vi "updateState.vi"(8 "error in (no error)":errorcluster, 10 "Monochromator in":refnum<class "Monochromator.lvclass">, 11 "SettingUpState in":refnum<class "SettingUpState.lvclass">) -> (0 "error out":errorcluster, 2 "Monochromator out":refnum<class "Monochromator.lvclass">, 3 "SettingUpState out":refnum<class "SettingUpState.lvclass">)   [LabVIEW 2016, in "SettingUpState.lvclass"]
uses:
  SettingUpState.lvclass
  Monochromator/Monochromator.lvclass
  Monochromator/Monochromator.lvclass/Monochromator.ctl
  Typedefs/SWStatus.ctl
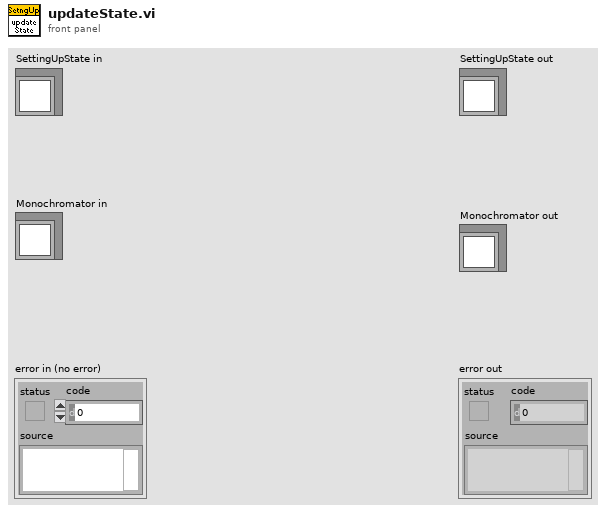
[diagram p1: front panel]
types:
  T1 = typedef "SWStatus.ctl" = enum16{"OfflineState", "ReadyState", "SettingUpState", "FaultState"}
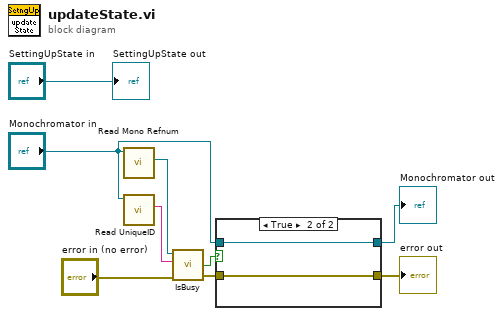
[diagram p0: block diagram]
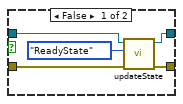
[diagram p2: hidden frame]
diagram:
  n1 = call "Read Mono Refnum.vi"("Monochromator in"="Monochromator in") -> ("Mono Refnum"=w3:refnum<k7>)  [unwired: 8 in, 2 out]
  n2 = call "Read UniqueID.vi"("Monochromator in"="Monochromator in") -> ("UniqueID"=w2:string)  [unwired: 8 in, 2 out]
  n3 = call "IsBusy.vi"("error in (no error)"="error in (no error)", "UniqueID"=w2, "RefNum In"=w3) -> ("error out"=w6:errorcluster, "IsBusy"=w7:bool)  [unwired: 1 in, 1 out]
  n4 = case shown="True" w7 {
    tunnel: [w10 w16] -> w5
    tunnel: w6 -> [w11 w16]
    tunnel: "Monochromator in" -> [w14 w15]
    tunnel: [w13 w15] -> w1
    frame False {
      n5 = call "updateState.vi"("error in (no error)"=w11, "SWStatus"=SWStatus."ReadyState", "Monochromator in"=w14) -> ("error out"=w10:errorcluster, "Monochromator out"=w13:refnum<class "Monochromator.lvclass">)  [unwired: 7 in]
    }
    frame True {
    }
  }
  "error out" <- w5
  "Monochromator out" <- w1
  "SettingUpState out" <- "SettingUpState in"
